vi "getOutCounterFileNameByMCSDB.vi"(10 "Entity":string) -> (2 "data":string)   [LabVIEW 2012]
uses:
  <vilib>/addons/database/Connection.llb/DB Tools Open Connec (Path).vi
  <vilib>/addons/database/Connection.llb/Conn Execute.vi
  <vilib>/addons/database/Recordset.llb/Rec Fetch String Data (R).vi
  <vilib>/addons/database/Recordset.llb/Rec Destroy - Connection.vi
  <vilib>/addons/database/NI_Database_API.lvlib
panel:
  out "concatenated string":string
  out "error out":errorcluster
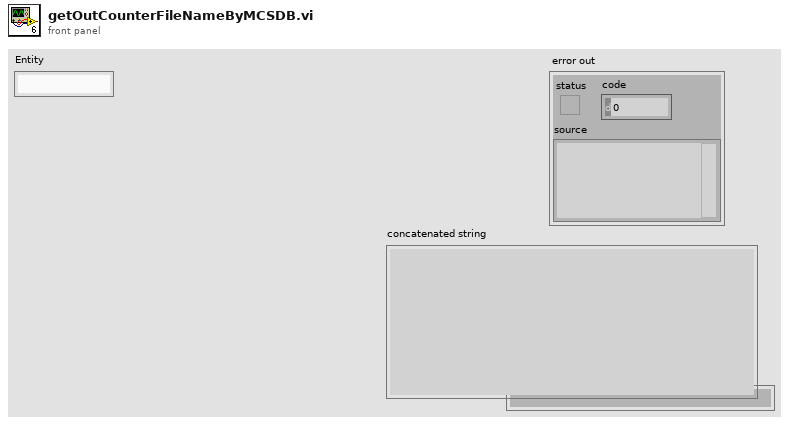
[diagram p1: front panel]
types:
  T1 = typedef "NI_Database_API.lvlib/Conn ObjectReference.ctl" = refnum<k1>
  T2 = typedef "NI_Database_API.lvlib/Rec ObjectReference.ctl" = refnum<k1>
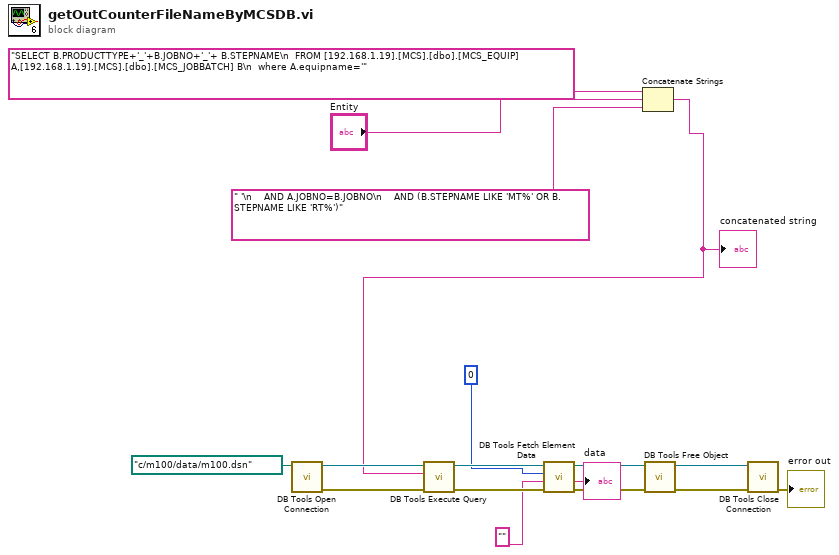
[diagram p0: block diagram]
diagram:
  n1 = call-poly <vilib>:"DB Tools Open Connection.vi"("connection information"=path "c:/m100/data/m100.dsn") -> ("error out"=w13:errorcluster, "connection reference"=w17:T1)  [unwired: 7 in]
  n2 = Concatenate Strings("SELECT B.PRODUCTTYPE+'_'+B.JOBNO+'_'+ B.STEPNAME\n  FROM [192.168.1.19].[MCS].[dbo].[MCS_EQUIP] A,[192.168.1.19].[MCS].[dbo].[MCS_JOBBATCH] B\n  where A.equipname='" ("string"), "Entity", " '\n    AND A.JOBNO=B.JOBNO\n    AND (B.STEPNAME LIKE 'MT%' OR B.STEPNAME LIKE 'RT%')" ("string")) -> (w1:string)
  "concatenated string" <- w1
  n3 = call-poly <vilib>:"DB Tools Execute Query.vi"("error in (no error)"=w13, "SQL query"=w1, "connection reference"=w17) -> ("error out"=w12:errorcluster, "recordset reference"=w16:T2)  [unwired: 5 in]
  n4 = call-poly <vilib>:"DB Tools Fetch Element Data.vi"("error in (no error)"=w12, "type"="", "column index"=0, "recordset reference"=w16) -> ("error out"=w11:errorcluster, "data"=→"data":string, "recordset reference out"=w15:T2)  [unwired: 3 in]
  n5 = call-poly <vilib>:"DB Tools Free Object.vi"("error in (no error)"=w11, "recordset reference"=w15) -> ("error out"=w10:errorcluster, "connection reference"=w14:T1)  [unwired: 8 in]
  n6 = call <vilib>:"DB Tools Close Connection.vi"("error in (no error)"=w10, "connection reference"=w14) -> ("error out"=→"error out":errorcluster)  [unwired: 5 in]
